vi "Begin.vi"(11 "Image Size":T1=enum."160x120") -> (0 "error out":errorcluster)   [LabVIEW 2012]
doc: "Called before other user functions, this VI is expected to open initial I/O refnums, load in file data, and do all program initialization. Notice that the <B>error out</B> terminal is simply used for data flow. Wiring it to other structures or subVIs ensures that this VI runs first."
uses:
  <vilib>/Rock Robotics/WPI/Camera/WPI_CameraImageSize.ctl
  <vilib>/Rock Robotics/SystemInterfaces/DIO/FPGA_DIOPWMChannel.ctl
  <vilib>/Rock Robotics/WPI/Joystick/WPI_JoystickDeviceEnum.ctl
  <vilib>/Rock Robotics/WPI/Camera/WPI_CameraWhite Balance Values.ctl
  <vilib>/Rock Robotics/WPI/Camera/WPI_CameraExposure Values.ctl
  <vilib>/Rock Robotics/WPI/Camera/WPI_CameraFrameRate.ctl
  <vilib>/Rock Robotics/SystemInterfaces/DIO/FPGA_DIORelayChannel.ctl
  <vilib>/Rock Robotics/SystemInterfaces/Typedef/FPGA_TypedefDigitalModule.ctl
  <vilib>/Rock Robotics/SystemInterfaces/DIO/FPGA_DIOChannel.ctl
  <vilib>/Rock Robotics/WPI/RobotDrive/WPI_RobotDriveOpen2MotorWithJaguar.vi
  <vilib>/Rock Robotics/WPI/MotorControl/WPI_MotorControlOpen Jaguar.vi
  <vilib>/Rock Robotics/WPI/MotorControl/WPI_MotorControlOpen Victor.vi
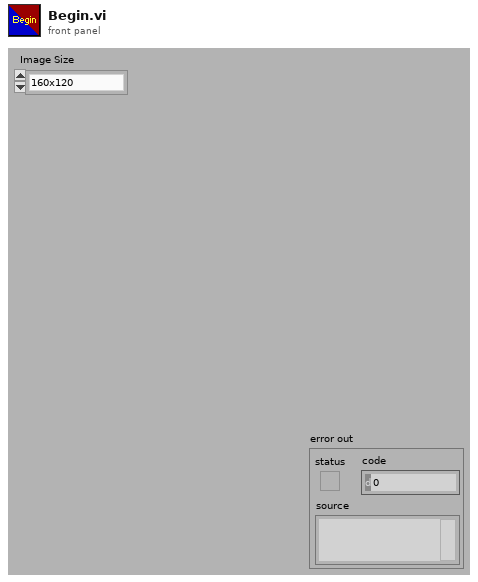
[diagram p1: front panel]
types:
  T1 = typedef "WPI_CameraImageSize.ctl" = enum16{"640x480", "320x240", "160x120"}
  T2 = typedef "FPGA_DIOPWMChannel.ctl" = enum8{"PWM 1", "PWM 2", "PWM 3", "PWM 4", "PWM 5", "PWM 6", "PWM 7", "PWM 8", "PWM 9", "PWM 10", "Invalid"}
  T3 = typedef "FPGA_DIOChannel.ctl" = enum8{"DIO 1", "DIO 2", "DIO 3", "DIO 4", "DIO 5", "DIO 6", "DIO 7", "DIO 8", "DIO 9", "DIO 10", "DIO 11", "DIO 12", "DIO 13", "DIO 14", "Invalid"}
  T4 = typedef "FPGA_DIORelayChannel.ctl" = enum8{"Relay 1", "Relay 2", "Relay 3", "Relay 4", "Relay 5", "Relay 6", "Relay 7", "Relay 8", "Invalid"}
  T5 = typedef "FPGA_TypedefDigitalModule.ctl" = enum16{"Digital Module 1", "Digital Module 2"}
  T6 = typedef "WPI_JoystickDeviceEnum.ctl" = enum16{"USB 1", "USB 2", "USB 3", "USB 4", "Kinect 1", "Kinect 2"}
  T7 = typedef "WPI_CameraFrameRate.ctl" = u32
  T8 = typedef "WPI_CameraExposure Values.ctl" = enum16{"Auto", "Flicker-free 50 Hz", "Flicker-free 60 Hz", "Hold current"}
  T9 = typedef "WPI_CameraWhite Balance Values.ctl" = enum16{"Auto", "Fixed indoor", "Fixed outdoor 1", "Fixed outdoor 2", "Fixed fluorescent 1", "Fixed fluorescent 2", "Hold current"}
  T10 = typedef "WPI_JoystickDevRef.ctl" = cluster{"Device":T6}
  T11 = typedef "WPI_RobotDriveDevRef.ctl" = cluster{"DevStatus":errorcluster, "Motors[]":T12[], "Square Inputs":bool, "Max Output":dbl, "Isochronous":bool}
  T12 = typedef "WPI_MotorControlDeviceRef.ctl" = cluster{"DeviceStatus":errorcluster, "Type":enum16{"PWM", "CAN"}, "PWM":cluster{"Digital Module":T5, "PWM Channel":T2, "DeadBand":T13}, "CAN":cluster{"Device Number":u8, "Control Mode":T14, "Semaphore":T15, "Max Vout":dbl}, "Invert":bool, "TransformRef":T16, "InvTransformRef":T16}
  T13 = typedef "WPI_PWMDeadband.ctl" = cluster{"Name":string, "maxPositivePwm":i32, "minPositivePwm":i32, "centerPwm":i32, "maxNegativePwm":i32, "minNegativePwm":i32, "angularRange":u16}
  T14 = typedef "WPI_CANJaguar_ControlMode.ctl" = enum8{"Percent VBus", "Current", "Speed", "Position", "Voltage"}
  T15 = typedef "Semaphore RefNum" = refnum<k1>
  T16 = typedef "WPI_PWMTransform_ConPane.ctl" = refnum<vi>
  T17 = typedef "WPI_ServoDeviceRef.ctl" = cluster{"DeviceStatus":errorcluster, "Digital Module":T5, "PWM Channel":T2, "DeadBand":T13}
  T18 = typedef "WPI_CameraDevRef.ctl" = cluster{"Camera Address":string, "CameraStatus":errorcluster, "Acquire Image Notifier":refnum<notifier>}
  T19 = typedef "WPI_RelayDevRef.ctl" = cluster{"DevStatus":errorcluster, "Relay Channel":T4, "Digital Module":T5, "Relay Direction":T20}
  T20 = typedef "WPI_RelayDirection.ctl" = enum16{"Both directions", "Forward only", "Reverse only"}
  T21 = typedef "WPI_DigitalInputDevRef.ctl" = cluster{"DevStatus":errorcluster, "DIO Channel":T3, "Digital Module":T5}
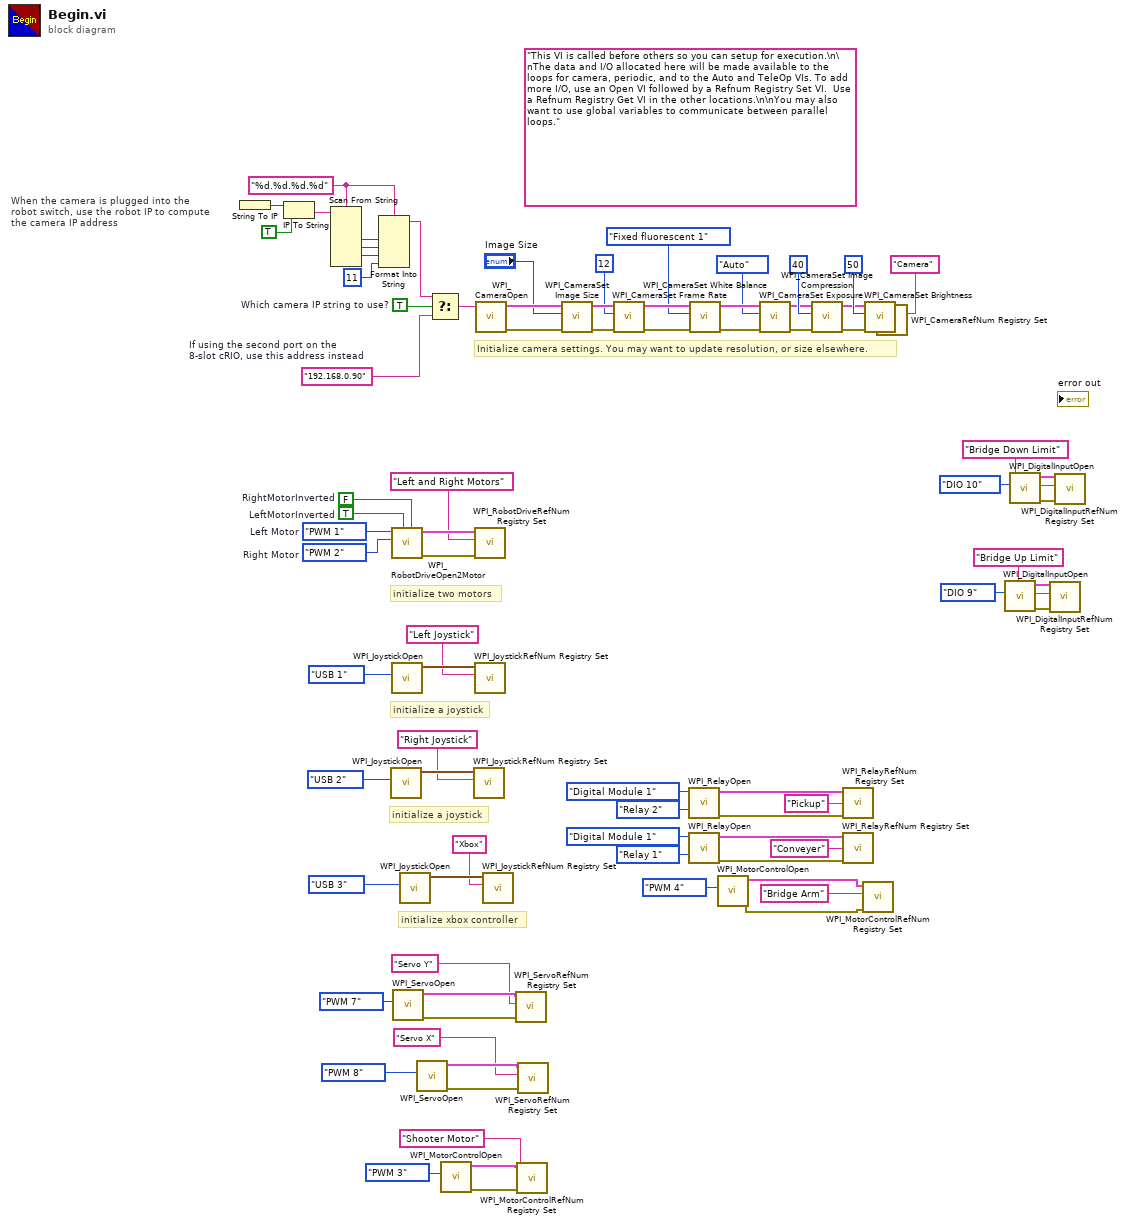
[diagram p0: block diagram]
diagram:
  w42 = TRUE  # Which camera IP string to use?
  w46 = "%d.%d.%d.%d" ("format string")
  (unwired) "This VI is called before others so you can setup for execution.\n\nThe data and I/O allocated here will be made available to the loops for camera, periodic, and to the Auto and TeleOp VIs. To add more I/O, use an Open VI followed by a Refnum Registry Set VI.  Use a Refnum Registry Get VI in the other locations.\n\nYou may also want to use global variables to communicate between parallel loops."
  w58 = FPGA_DIOPWMChannel."PWM 2"  # Right Motor
  w59 = FPGA_DIOPWMChannel."PWM 1"  # Left Motor
  w43 = "192.168.0.90"  # If using the second port on the 8-slot cRIO, use this address instead
  w82 = TRUE  # LeftMotorInverted
  w83 = FALSE  # RightMotorInverted
  # "initialize xbox controller"
  # "initialize a joystick"
  # "When the camera is plugged into the\nrobot switch, use the robot IP to compute\nthe camera IP address"
  # "initialize a joystick"
  # "initialize two motors"
  # "Initialize camera settings. You may want to update resolution, or size elsewhere."
  n1 = String To IP() -> (0:w53:u32)  [unwired: 1 in]
  n2 = IP To String(1:TRUE ("dot notation? (F)"), 2:w53) -> (0:w51:string)
  n3 = Scan From String(format string=w46, input string=w51) -> (output 1=w50:i32, output 2=w49:i32, output 3=w48:i32)  [unwired: 7 in, 3 out]
  n4 = Format Into String(format string=w46, w50, w49, w48, 11 ("Compression")) -> (resulting string=w44:string)  [unwired: 2 in, 1 out]
  n5 = call <vilib>:"WPI_JoystickOpen.vi"("JoystickDevice"=WPI_JoystickDeviceEnum."USB 2") -> ("JoystickDevRef"=w40:T10)  [unwired: 10 out]
  n6 = call-poly <vilib>:"WPI_RobotDriveOpen2Motor.vi"("Right Motor Inverted"=w83, "Left Motor Inverted"=w82, "Right Motor"=w58, "Left Motor"=w59) -> ("error out"=w77:errorcluster, "RobotDriveDevRef"=w80:T11)  [unwired: 1 in, 5 out]
  n7 = call <vilib>:"WPI_JoystickOpen.vi"("JoystickDevice"=WPI_JoystickDeviceEnum."USB 1") -> ("JoystickDevRef"=w79:T10)  [unwired: 10 out]
  n8 = call <vilib>:"WPI_ServoOpen.vi"("PWM Channel"=FPGA_DIOPWMChannel."PWM 7") -> ("error out"=w32:errorcluster, "ServoDeviceRef"=w33:T17)  [unwired: 9 in]
  n9 = call <vilib>:"WPI_JoystickOpen.vi"("JoystickDevice"=WPI_JoystickDeviceEnum."USB 3") -> ("JoystickDevRef"=w25:T10)  [unwired: 10 out]
  n10 = call <vilib>:"WPI_ServoOpen.vi"("PWM Channel"=FPGA_DIOPWMChannel."PWM 8") -> ("error out"=w29:errorcluster, "ServoDeviceRef"=w30:T17)  [unwired: 9 in]
  n11 = Select(t=w44, s=w42, f=w43) -> (s? t:f=w45:string)
  n12 = call-poly <vilib>:"WPI_MotorControlOpen.vi"("PWM Channel"=FPGA_DIOPWMChannel."PWM 3") -> ("error out"=w36:errorcluster, "MotorControlDeviceRef"=w37:T12)  [unwired: 9 in]
  n13 = call <vilib>:"WPI_JoystickRefNum Registry Set.vi"("refnum name"="Right Joystick", "JoystickDevRef"=w40) -> ()  [unwired: 1 in, 9 out]
  n14 = call <vilib>:"WPI_RobotDriveRefNum Registry Set.vi"("error in (no error)"=w77, "refnum name"="Left and Right Motors", "RobotDriveDevRef"=w80) -> ()  [unwired: 9 out]
  n15 = call <vilib>:"WPI_JoystickRefNum Registry Set.vi"("refnum name"="Left Joystick", "JoystickDevRef"=w79) -> ()  [unwired: 1 in, 9 out]
  n16 = call <vilib>:"WPI_CameraOpen.vi"("Camera Address"=w45) -> ("error out"=w68:errorcluster, "CameraDevRef"=w69:T18)  [unwired: 1 in, 8 out]
  n17 = call <vilib>:"WPI_JoystickRefNum Registry Set.vi"("refnum name"="Xbox", "JoystickDevRef"=w25) -> ()  [unwired: 1 in, 9 out]
  n18 = call <vilib>:"WPI_ServoRefNum Registry Set.vi"("error in (no error)"=w32, "refnum name"="Servo Y", "ServoDeviceRef"=w33) -> ()  [unwired: 7 in, 2 out]
  n19 = call <vilib>:"WPI_MotorControlRefNum Registry Set.vi"("error in (no error)"=w36, "refnum name"="Shooter Motor", "MotorControlDevRef"=w37) -> ()  [unwired: 7 in, 2 out]
  n20 = call <vilib>:"WPI_ServoRefNum Registry Set.vi"("error in (no error)"=w29, "refnum name"="Servo X", "ServoDeviceRef"=w30) -> ()  [unwired: 7 in, 2 out]
  n21 = call <vilib>:"WPI_CameraSet Image Size.vi"("error in (no error)"=w68, "Image Size"="Image Size", "CameraDevRef"=w69) -> ("error out"=w67:errorcluster, "CameraDevRef Out"=w70:T18)  [unwired: 7 out]
  n22 = call <vilib>:"WPI_CameraSet Frame Rate.vi"("error in (no error)"=w67, "Frame Rate (fps)"=T7 12, "CameraDevRef"=w70) -> ("error out"=w66:errorcluster, "CameraDevRef Out"=w72:T18)  [unwired: 7 out]
  n23 = call <vilib>:"WPI_RelayOpen.vi"("Relay Channel"=FPGA_DIORelayChannel."Relay 2", "Digital Module (Module 1)"=FPGA_TypedefDigitalModule."Digital Module 1") -> ("error out"=w22:errorcluster, "RelayDevRef"=w21:T19)  [unwired: 8 in]
  n24 = call <vilib>:"WPI_RelayOpen.vi"("Relay Channel"=FPGA_DIORelayChannel."Relay 1", "Digital Module (Module 1)"=FPGA_TypedefDigitalModule."Digital Module 1") -> ("error out"=w17:errorcluster, "RelayDevRef"=w16:T19)  [unwired: 8 in]
  n25 = call <vilib>:"WPI_CameraSet White Balance.vi"("error in (no error)"=w66, "White Balance"=WPI_CameraWhite_Balance_Values."Fixed fluorescent 1", "CameraDevRef"=w72) -> ("error out"=w65:errorcluster, "CameraDevRef Out"=w71:T18)  [unwired: 7 out]
  n26 = call-poly <vilib>:"WPI_MotorControlOpen.vi"("PWM Channel"=FPGA_DIOPWMChannel."PWM 4") -> ("error out"=w4:errorcluster, "MotorControlDeviceRef"=w1:T12)  [unwired: 9 in]
  n27 = call <vilib>:"WPI_CameraSet Exposure.vi"("error in (no error)"=w65, "Exposure"=WPI_CameraExposure_Values."Auto", "CameraDevRef"=w71) -> ("error out"=w64:errorcluster, "CameraDevRef Out"=w74:T18)  [unwired: 7 out]
  n28 = call <vilib>:"WPI_CameraSet Image Compression.vi"("error in (no error)"=w64, "Compression"=40, "CameraDevRef"=w74) -> ("error out"=w63:errorcluster, "CameraDevRef Out"=w73:T18)  [unwired: 7 out]
  n29 = call <vilib>:"WPI_RelayRefNum Registry Set.vi"("error in (no error)"=w22, "refnum name"="Pickup", "RelayDevRef"=w21) -> ()  [unwired: 7 in, 2 out]
  n30 = call <vilib>:"WPI_RelayRefNum Registry Set.vi"("error in (no error)"=w17, "refnum name"="Conveyer", "RelayDevRef"=w16) -> ()  [unwired: 7 in, 2 out]
  n31 = call <vilib>:"WPI_MotorControlRefNum Registry Set.vi"("error in (no error)"=w4, "refnum name"="Bridge Arm", "MotorControlDevRef"=w1) -> ()  [unwired: 7 in, 2 out]
  n32 = call <vilib>:"WPI_CameraSet Brightness.vi"("error in (no error)"=w63, "Brightness"=50, "CameraDevRef"=w73) -> ("error out"=w61:errorcluster, "CameraDevRef Out"=w62:T18)  [unwired: 7 out]
  n33 = call <vilib>:"WPI_CameraRefNum Registry Set.vi"("error in (no error)"=w61, "refnum name"="Camera", "CameraDevRef"=w62) -> ()  [unwired: 9 out]
  n34 = call <vilib>:"WPI_DigitalInputOpen.vi"("DIO Channel"=FPGA_DIOChannel."DIO 9") -> ("error out"=w8:errorcluster, "DigitalInputDevRef"=w7:T21)  [unwired: 9 in]
  n35 = call <vilib>:"WPI_DigitalInputOpen.vi"("DIO Channel"=FPGA_DIOChannel."DIO 10") -> ("error out"=w12:errorcluster, "DigitalInputDevRef"=w11:T21)  [unwired: 9 in]
  n36 = call <vilib>:"WPI_DigitalInputRefNum Registry Set.vi"("error in (no error)"=w8, "refnum name"="Bridge Up Limit", "DigitalInputDevRef"=w7) -> ()  [unwired: 7 in, 2 out]
  n37 = call <vilib>:"WPI_DigitalInputRefNum Registry Set.vi"("error in (no error)"=w12, "refnum name"="Bridge Down Limit", "DigitalInputDevRef"=w11) -> ()  [unwired: 7 in, 2 out]
